vi "Autonomous Independent (2).vi"   [LabVIEW 2015]
doc: "This VI is called when autonomous begins, and will automatically be terminated when autonomous ends. You can carry out timed or sensor driven robot movement independently without needing to return to the caller."
uses:
  <vilib>/Rock Robotics/WPI/RobotDrive/WPI_RobotDriveArcadeDrive_Standard(NoSaturation).vi
  <vilib>/Rock Robotics/Network Tables/NT Write Numeric Array.vi
panel:
  # "Be sure to right-click and choose Data Operations>>Make Current Value default if you want to save the array values with the VI"
types:
  T1 = typedef "WPI_JoystickDevRef.ctl" = cluster{"Device":T2}
  T2 = typedef "WPI_JoystickDeviceEnum.ctl" = enum16{"USB 0", "USB 1", "USB 2", "USB 3", "USB 4", "USB 5"}
  T3 = typedef "WPI_DigitalInputDevRef.ctl" = cluster{"DevStatus":errorcluster, "DIO Channel":T4}
  T4 = typedef "FPGA_DIOChannel.ctl" = enum8{"DIO 0", "DIO 1", "DIO 2", "DIO 3", "DIO 4", "DIO 5", "DIO 6", "DIO 7", "DIO 8", "DIO 9", "DIO MXP 0", "DIO MXP 1", "DIO MXP 2", "DIO MXP 3", "DIO MXP 4", "DIO MXP 5", "DIO MXP 6", "DIO MXP 7", "DIO MXP 8", "DIO MXP 9", "DIO MXP 10", "DIO MXP 11", "DIO MXP 12", "DIO MXP 13", "DIO MXP 14", "DIO MXP 15", "Invalid"}
  T5 = typedef "WPI_MotorControlDeviceRef.ctl" = cluster{"DeviceStatus":errorcluster, "Type":T6, "PWM":cluster{"PWM Channel":T7, "DeadBand":T8}, "CAN":cluster{"Device Number":u8, "Control Mode":T9, "Semaphore":T10, "Max Vout":dbl, "TalonSRX Control Mode":T11}, "Invert":bool}
  T6 = typedef "WPI_MotorControlType.ctl" = enum16{"PWM", "CAN", "CANTalonSRX"}
  T7 = typedef "FPGA_DIOPWMChannel.ctl" = enum8{"PWM 0", "PWM 1", "PWM 2", "PWM 3", "PWM 4", "PWM 5", "PWM 6", "PWM 7", "PWM 8", "PWM 9", "PWM MXP 0", "PWM MXP 1", "PWM MXP 2", "PWM MXP 3", "PWM MXP 4", "PWM MXP 5", "PWM MXP 6", "PWM MXP 7", "PWM MXP 8", "PWM MXP 9", "Invalid"}
  T8 = typedef "WPI_PWMDeadband.ctl" = cluster{"Name":string, "maxPositivePwm":i32, "minPositivePwm":i32, "centerPwm":i32, "maxNegativePwm":i32, "minNegativePwm":i32, "angularRange":u16}
  T9 = typedef "WPI_CANJaguar_ControlMode.ctl" = enum8{"Percent VBus", "Current", "Speed", "Position", "Voltage"}
  T10 = typedef "Semaphore RefNum" = refnum<k1>
  T11 = typedef "WPI_CANTalonSRX_APIControlMode.ctl" = enum8{"Percent VBus", "Speed", "Position", "Slave", "Unchanged / Invalid", "Voltage Compensation", "Current", "Motion Profile"}
  T12 = typedef "WPI_GyroDevRef.ctl" = cluster{"DevStatus":errorcluster, "Analog Channel":T13, "Offset":dbl, "Gain (VoltsPerDegree/Second)":dbl, "Gyro Type":enum16{"Analog", "XRS450"}, "Handle":i32, "SPI Bus":T14, "Device Found":bool, "Sample Rate":dbl, "Calibrate On Open":bool}
  T13 = typedef "FPGA_AIChannel.ctl" = enum8{"AI 0", "AI 1", "AI 2", "AI 3", "AI MXP 0", "AI MXP 1", "AI MXP 2", "AI MXP 3", "Invalid"}
  T14 = typedef "spi_bus.ctl" = enum16{"SPI On-Board, CS0", "SPI On-Board, CS1", "SPI On-Board, CS2", "SPI On-Board, CS3", "SPI MXP", "Invalid"}
  T15 = typedef "WPI_CameraDevRef.ctl" = cluster{"Camera Address":string, "CameraStatus":errorcluster}
  T16 = typedef "WPI_AccelerometerDevRef.ctl" = cluster{"DevStatus":errorcluster, "Scaling":T17, "Analog Channels":T18, "I2C Bus":T19, "SPI Bus":T14, "Accel Range":T20, "ADXL Axes":T21, "Handle":i32, "Device Address":u8, "Accel Type":enum16{"Analog", "ADXL345 I2C", "ADXL345 SPI", "Internal", "ADXL362 SPI"}}
  T17 = typedef "WPI_AccelerometerScaling.ctl" = cluster{"Gain (VoltsPerG)":dbl, "Center Voltage":dbl}
  T18 = typedef "WPI_AccelerometerAnalogChannels.ctl" = cluster{"X-Axis":T13, "Y-Axis":T13, "Z-Axis":T13}
  T19 = typedef "i2c_bus.ctl" = enum16{"I2C On-Board", "I2C MXP", "Invalid"}
  T20 = typedef "ADXL345 Range.ctl" = u8
  T21 = typedef "WPI_AccelerometerADXL345 Axes.ctl" = cluster{"X-Axis":bool, "Y-Axis":bool, "Z-Axis":bool}
  T22 = typedef "WPI_EncoderDevRef.ctl" = cluster{"DevStatus":errorcluster, "EncoderIndex":T23, "CounterIndex":T24, "DistancePerCount":dbl, "Decoding Type":T25}
  T23 = typedef "FPGA_EncoderIdx.ctl" = enum8{"Enc 0", "Enc 1", "Enc 2", "Enc 3", "Enc 4", "Enc 5", "Enc 6", "Enc 7", "Invalid"}
  T24 = typedef "FPGA_CounterCtrSystemIndex.ctl" = enum8{"Ctr 0", "Ctr 1", "Ctr 2", "Ctr 3", "Ctr 4", "Ctr 5", "Ctr 6", "Ctr 7", "Invalid"}
  T25 = typedef "WPI_EncoderType.ctl" = enum16{"1x", "2x", "4x"}
  T26 = typedef "WPI_RobotDriveDevRef.ctl" = cluster{"DevStatus":errorcluster, "Motors[]":T5[], "Square Inputs":bool, "Max Output":dbl}
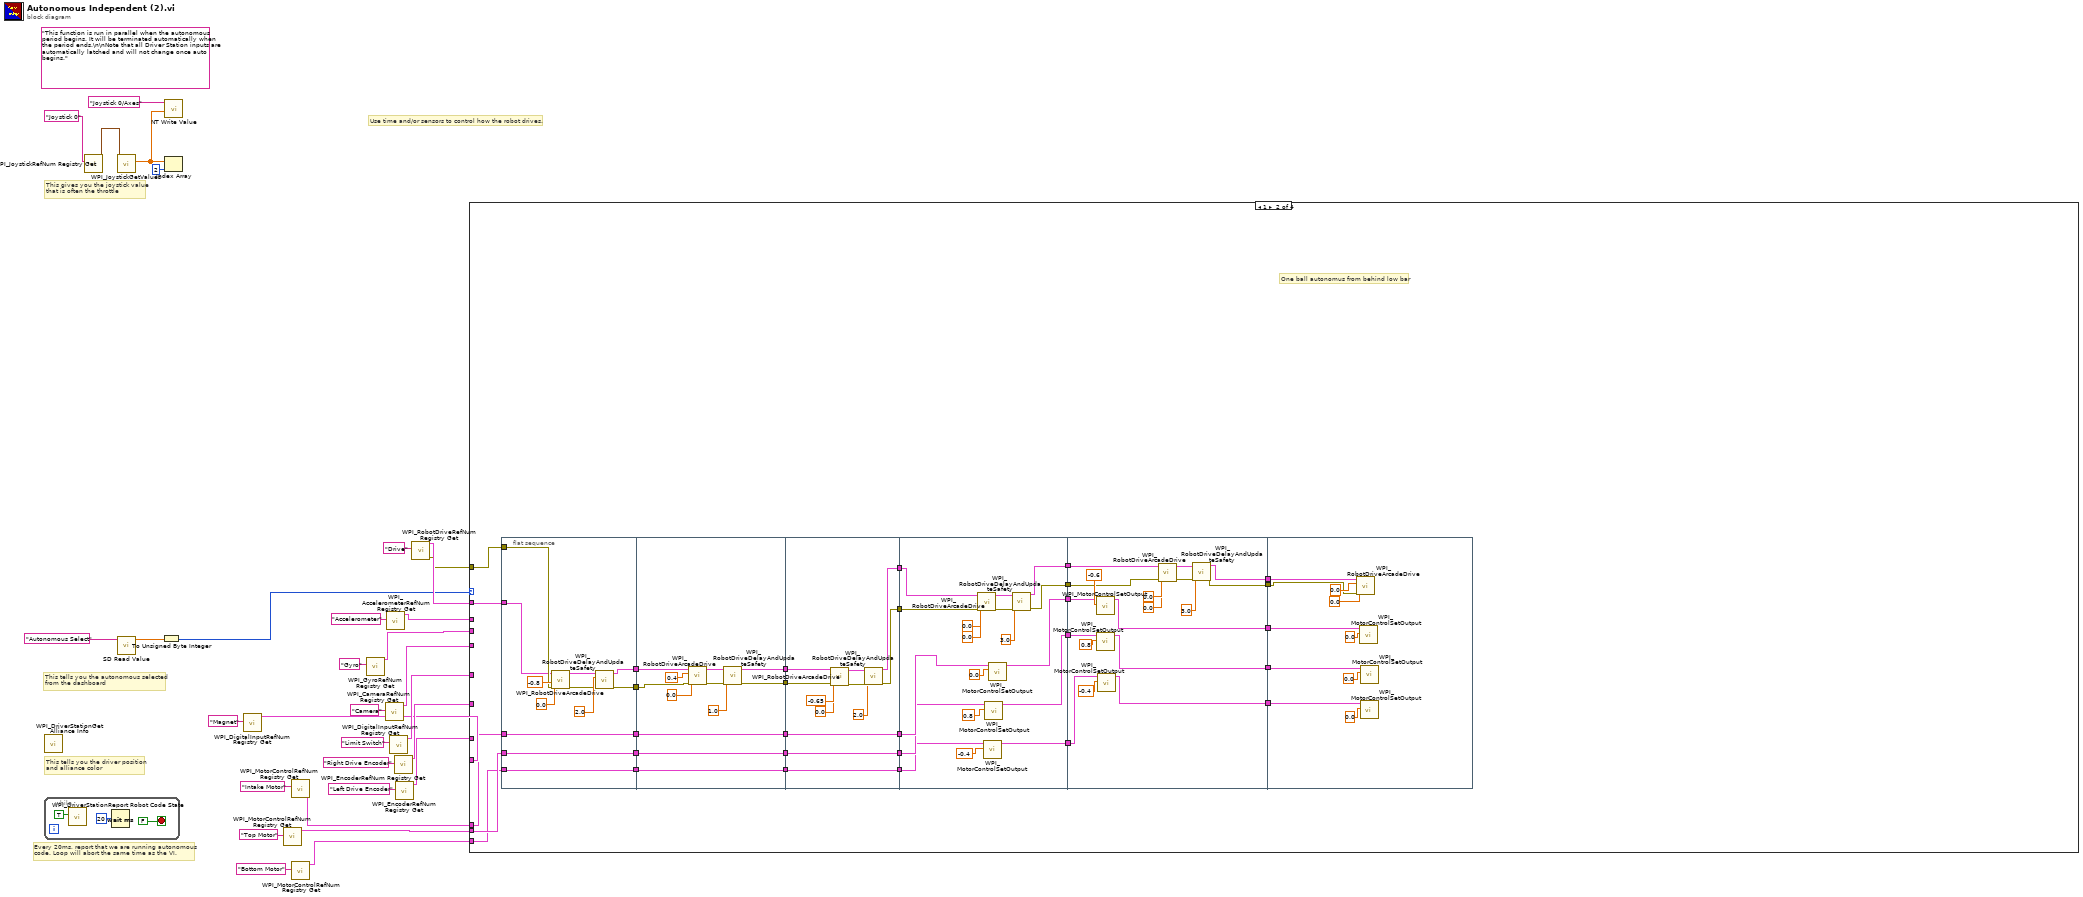
[diagram p0: block diagram]
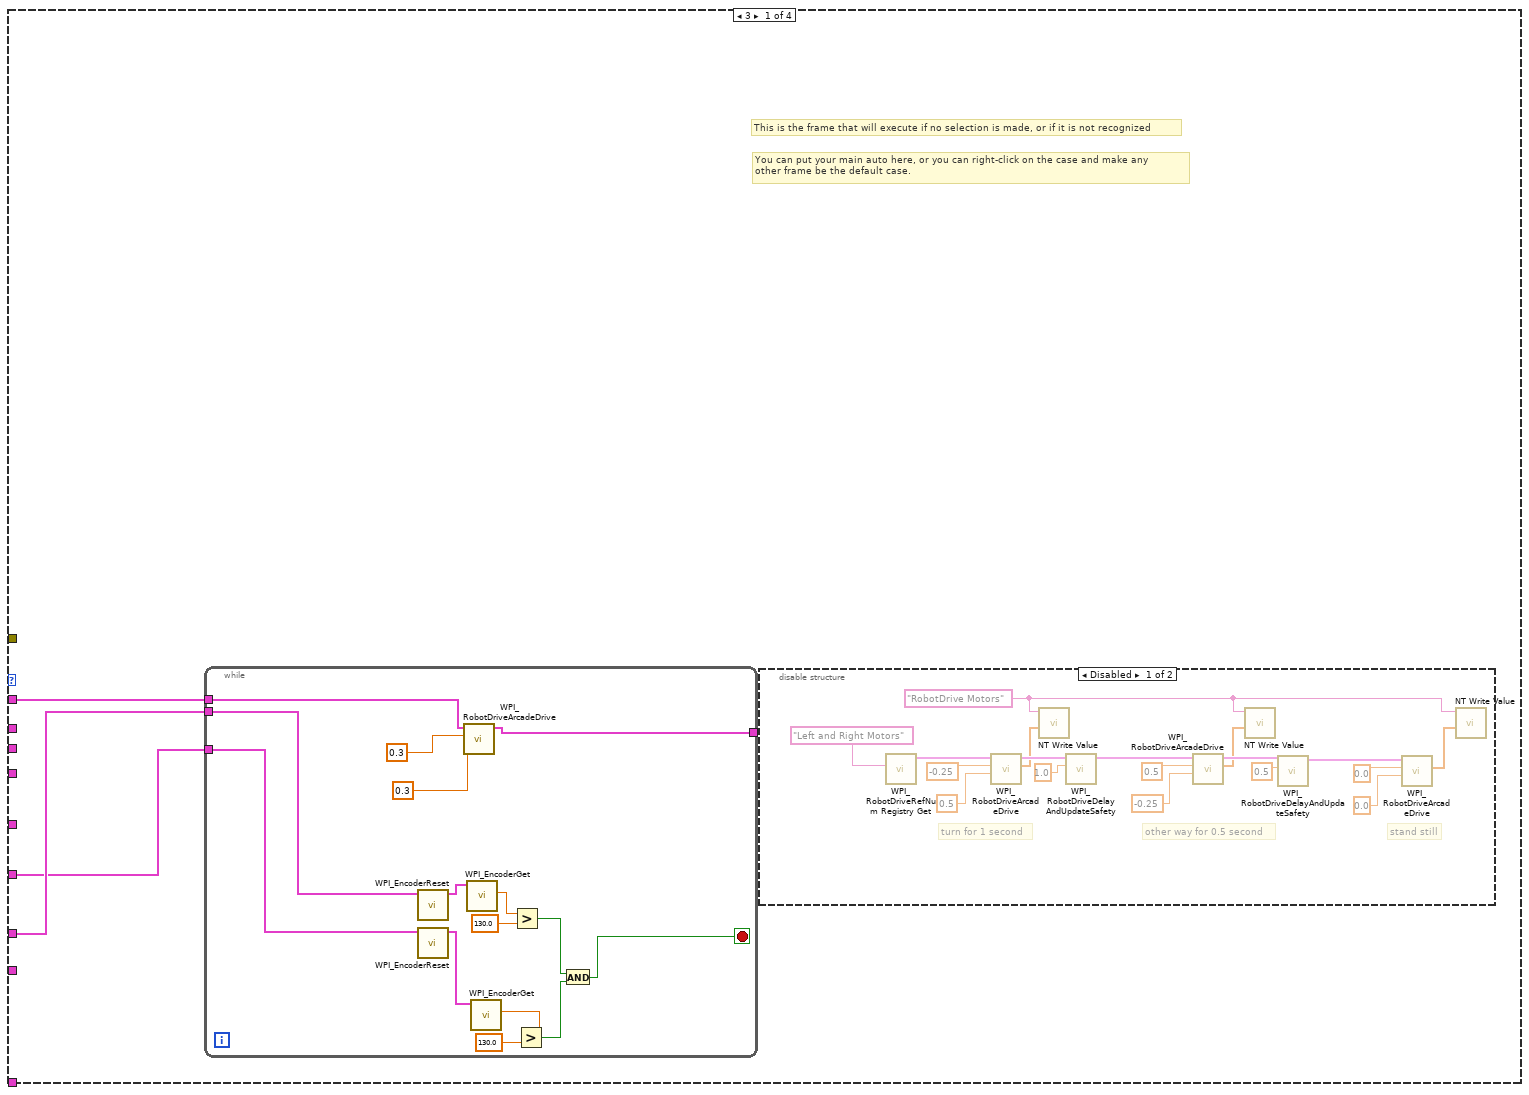
[diagram p2: hidden frame]
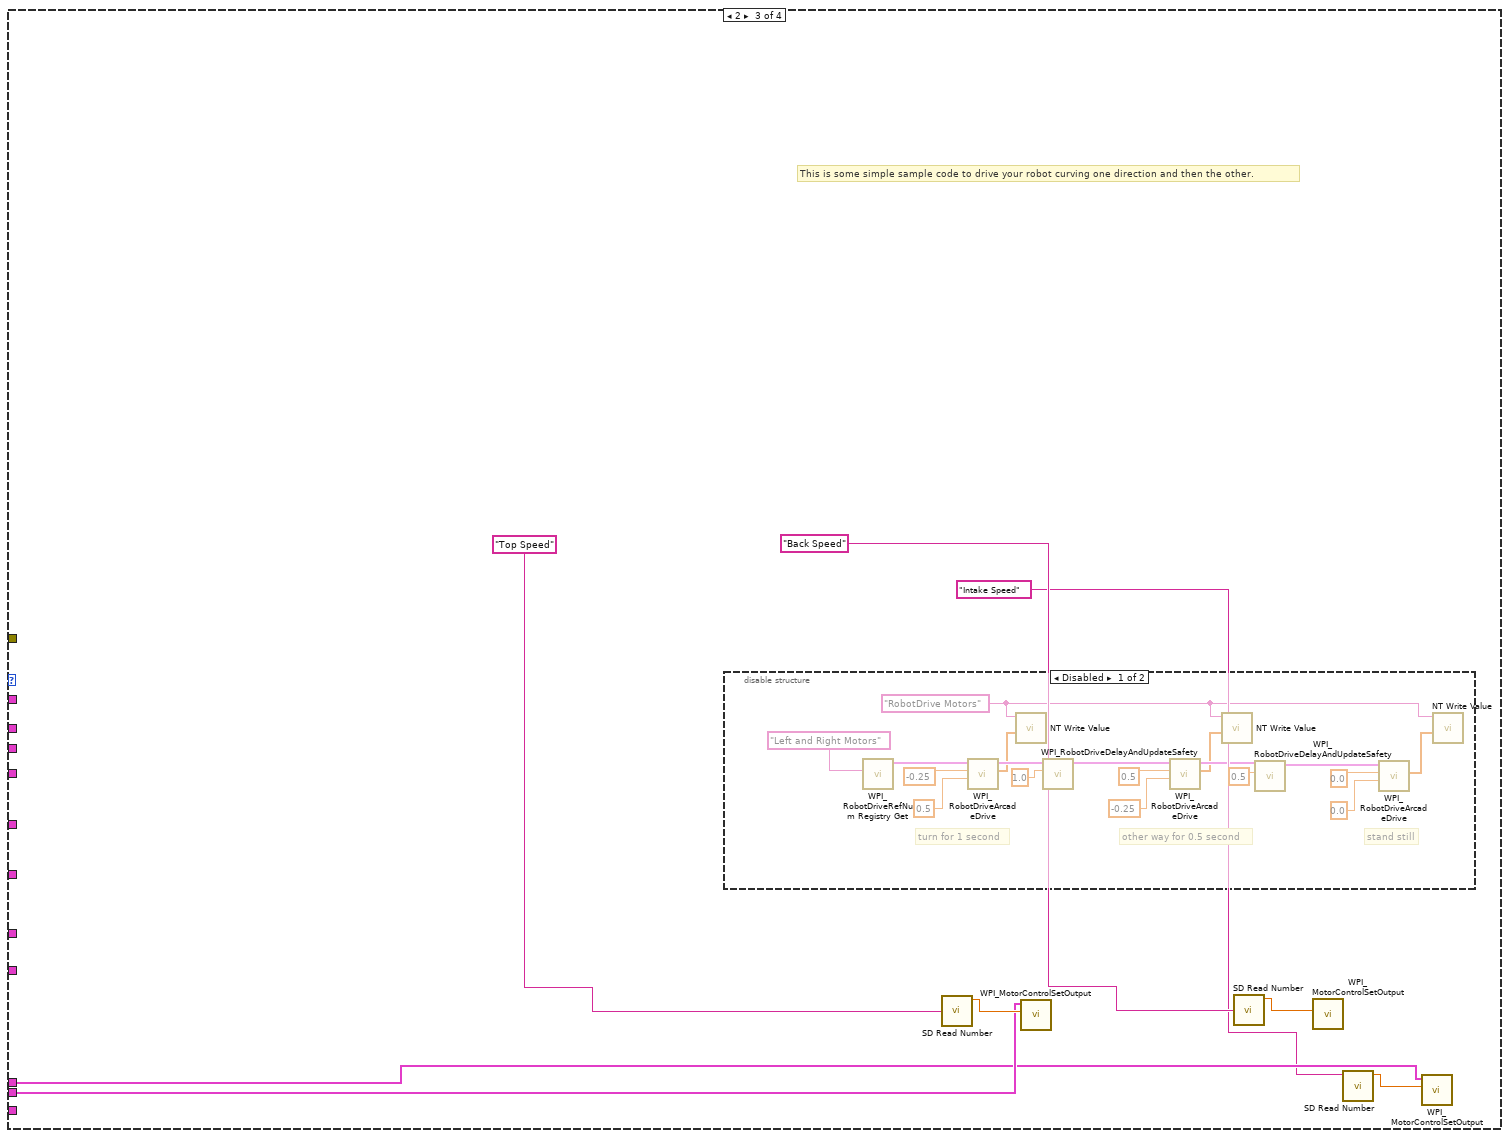
[diagram p4: hidden frame]
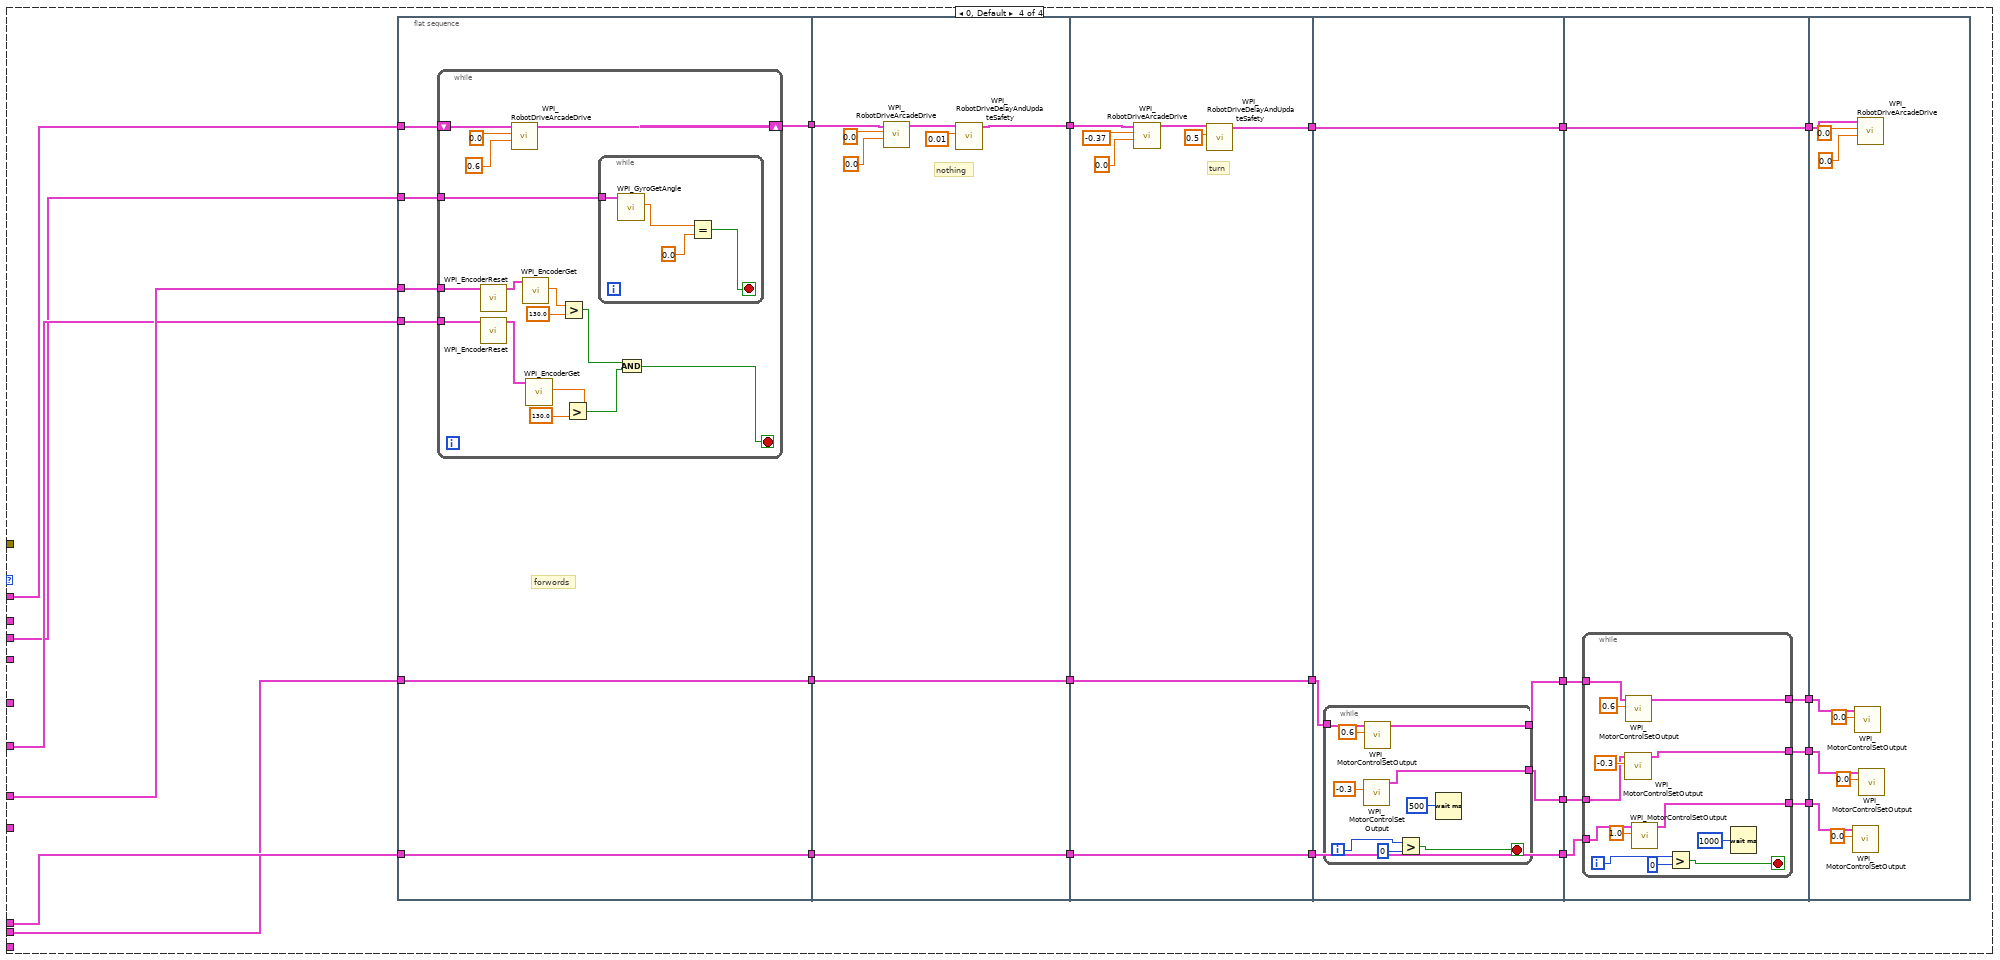
[diagram p6: hidden frame]
diagram:
  (unwired) "This function is run in parallel when the autonomous period begins. It will be terminated automatically when the period ends.\n\nNote that all Driver Station inputs are automatically latched and will not change once auto begins."
  # "This tells you the autonomous selected\nfrom the dashboard"
  # "Every 20ms, report that we are running autonomous\ncode. Loop will abort the same time as the VI."
  # "This tells you the driver position\nand alliance color"
  # "Use time and/or sensors to control how the robot drives."
  # "This gives you the joystick value\nthat is often the throttle"
  n1 = while {
    stop <- FALSE stop-if-true
    n2 = call <vilib>:"WPI_DriverStationReport Robot Code State.vi"("Autonomous"=TRUE) -> ()  [unwired: 10 in, 1 out]
    n3 = Wait (ms)(milliseconds to wait=u32 20) -> ()  [unwired: 1 out]
  }
  n4 = call <vilib>:"WPI_DriverStationGet Alliance Info.vi"() -> ()  [unwired: 12 out]
  n5 = call <vilib>:"WPI_JoystickRefNum Registry Get.vi"("refnum name"="Joystick 0") -> ("JoystickDevRef"=w30:T1)  [unwired: 1 in, 9 out]
  n6 = call <vilib>:"WPI_JoystickGetValues.vi"("JoystickDevRef"=w30) -> ("Axes"=w28:dbl[])  [unwired: 6 in, 4 out]
  n7 = call-poly <vilib>:"SD Read Value.vi"("Name"="Autonomous Select") -> ("Numeric"=w16:dbl)  [unwired: 8 in, 2 out]
  n8 = To Unsigned Byte Integer(number=w16) -> (unsigned 8bit integer=w14:u8)
  n9 = call-poly <vilib>:"NT Write Value.vi"("Numeric Array"=w28, "Name"="Joystick 0/Axes") -> ()  [unwired: 9 in, 1 out]
  n10 = Index Array(array=w28, index=2) -> ()  [unwired: 1 out]
  n11 = call <vilib>:"WPI_DigitalInputRefNum Registry Get.vi"("refnum name"="Magnet") -> ("DigitalInputDevRef"=w17:T3)  [unwired: 9 in, 1 out]
  n12 = call <vilib>:"WPI_MotorControlRefNum Registry Get.vi"("refnum name"="Top Motor") -> ("MotorControlDevRef"=w3:T5)  [unwired: 9 in, 1 out]
  n13 = call <vilib>:"WPI_MotorControlRefNum Registry Get.vi"("refnum name"="Intake Motor") -> ("MotorControlDevRef"=w11:T5)  [unwired: 9 in, 1 out]
  n14 = call <vilib>:"WPI_MotorControlRefNum Registry Get.vi"("refnum name"="Bottom Motor") -> ("MotorControlDevRef"=w1:T5)  [unwired: 9 in, 1 out]
  n15 = call <vilib>:"WPI_GyroRefNum Registry Get.vi"("refnum name"="Gyro") -> ("GyroDevRef"=w22:T12)  [unwired: 9 in, 1 out]
  n16 = call <vilib>:"WPI_CameraRefNum Registry Get.vi"("refnum name"="Camera") -> ("CameraDevRef"=w21:T15)  [unwired: 9 in, 1 out]
  n17 = call <vilib>:"WPI_AccelerometerRefNum Registry Get.vi"("refnum name"="Accelerometer") -> ("AccelerometerDevRef"=w23:T16)  [unwired: 9 in, 1 out]
  n18 = call <vilib>:"WPI_DigitalInputRefNum Registry Get.vi"("refnum name"="Limit Switch") -> ("DigitalInputDevRef"=w20:T3)  [unwired: 9 in, 1 out]
  n19 = call <vilib>:"WPI_EncoderRefNum Registry Get.vi"("refnum name"="Right Drive Encoder") -> ("EncoderDevRef"=w19:T22)  [unwired: 9 in, 1 out]
  n20 = call <vilib>:"WPI_EncoderRefNum Registry Get.vi"("refnum name"="Left Drive Encoder") -> ("EncoderDevRef"=w18:T22)  [unwired: 9 in, 1 out]
  n21 = call <vilib>:"WPI_RobotDriveRefNum Registry Get.vi"("refnum name"="Drive") -> ("error out"=w2:errorcluster, "RobotDriveDevRef"=w26:T26)  [unwired: 9 in]
  n22 = case shown="1" w14 {
    tunnel: w26 -> [w35 w83 _ w213]
    tunnel: w23 -> [_ _ _ _]
    tunnel: w22 -> [_ _ _ w209]
    tunnel: w21 -> [_ _ _ _]
    tunnel: w20 -> [_ _ _ _]
    tunnel: w19 -> [w36 _ _ w210]
    tunnel: w18 -> [w37 _ _ w211]
    tunnel: w17 -> [_ _ _ _]
    tunnel: w3 -> [_ w78 w188 w214]
    tunnel: w11 -> [_ w82 w185 w215]
    tunnel: w2 -> [_ w85 _ _]
    tunnel: w1 -> [_ w71 _ _]
    frame 3 {
      # "You can put your main auto here, or you can right-click on the case and make any\nother frame be the default case."
      # "This is the frame that will execute if no selection is made, or if it is not recognized"
      n23 = while {
        tunnel: w37 -> [w46]
        tunnel: w36 -> [w45]
        tunnel: w35 -> [w41]
        tunnel: [w40] -> _
        stop <- w42 stop-if-true
        n24 = call <vilib>:"WPI_EncoderReset.vi"("EncoderDevRef"=w46) -> ("EncoderDevRef"=w48:T22)  [unwired: 9 in, 1 out]
        n25 = call <vilib>:"WPI_EncoderReset.vi"("EncoderDevRef"=w45) -> ("EncoderDevRef"=w52:T22)  [unwired: 9 in, 1 out]
        n26 = call-poly <vilib>:"WPI_RobotDriveArcadeDrive.vi"("Y axis value"=0.3, "X axis value"=0.3, "RobotDriveDevRef"=w41) -> ("RobotDriveDevRef"=w40:T26)  [unwired: 6 in, 2 out]
        n27 = call <vilib>:"WPI_EncoderGet.vi"("EncoderDevRef"=w48) -> ("Distance"=w49:dbl)  [unwired: 5 in, 5 out]
        n28 = call <vilib>:"WPI_EncoderGet.vi"("EncoderDevRef"=w52) -> ("Distance"=w51:dbl)  [unwired: 5 in, 5 out]
        n29 = Greater?(x=w49, y=130.0) -> (0:w44:bool)
        n30 = Greater?(x=w51, y=130.0) -> (0:w43:bool)
        n31 = And(x=w44, y=w43) -> (x .and. y?=w42:bool)
      }
      n32 = disable-structure shown="Disabled" {
        frame Disabled {
          w54 = "RobotDrive Motors" ("Name")
          # "stand still"
          # "other way for 0.5 second"
          # "turn for 1 second"
          n33 = call <vilib>:"WPI_RobotDriveRefNum Registry Get.vi"("refnum name"="Left and Right Motors") -> ("RobotDriveDevRef"=w70:T26)  [unwired: 1 in, 9 out]
          n34 = call-poly <vilib>:"WPI_RobotDriveArcadeDrive.vi"("Y axis value"=0.5 ("X axis value"), "X axis value"=-0.25, "RobotDriveDevRef"=w70) -> ("Motor Values"=w53:dbl[], "RobotDriveDevRef"=w63:T26)  [unwired: 1 in, 6 out]
          n35 = call-poly <vilib>:"NT Write Value.vi"("Numeric Array"=w53, "Name"=w54) -> ()  [unwired: 9 in, 1 out]
          n36 = call <vilib>:"WPI_RobotDriveDelayAndUpdateSafety.vi"("Delay (s)"=1.0, "RobotDriveDevRef"=w63) -> ("RobotDriveDevRef 2"=w64:T26)  [unwired: 8 in, 1 out]
          n37 = call-poly <vilib>:"WPI_RobotDriveArcadeDrive.vi"("Y axis value"=-0.25 ("X axis value"), "X axis value"=0.5, "RobotDriveDevRef"=w64) -> ("Motor Values"=w55:dbl[], "RobotDriveDevRef"=w65:T26)  [unwired: 1 in, 6 out]
          n38 = call-poly <vilib>:"NT Write Value.vi"("Numeric Array"=w55, "Name"=w54) -> ()  [unwired: 9 in, 1 out]
          n39 = call <vilib>:"WPI_RobotDriveDelayAndUpdateSafety.vi"("Delay (s)"=0.5, "RobotDriveDevRef"=w65) -> ("RobotDriveDevRef 2"=w66:T26)  [unwired: 8 in, 1 out]
          n40 = call-poly <vilib>:"WPI_RobotDriveArcadeDrive.vi"("Y axis value"=0.0 ("X axis value"), "X axis value"=0.0, "RobotDriveDevRef"=w66) -> ("Motor Values"=w56:dbl[])  [unwired: 1 in, 7 out]
          n41 = call-poly <vilib>:"NT Write Value.vi"("Numeric Array"=w56, "Name"=w54) -> ()  [unwired: 9 in, 1 out]
        }
        frame Enabled {
        }
      }
    }
    frame 1 {
      # "One ball autonomus from behind low bar"
      n42 = flat-sequence {
        tunnel: [w107] -> w100
        tunnel: [w106] -> w86
        tunnel: w85 -> [w105]
        tunnel: w83 -> [w104]
        tunnel: w82 -> [w103]
        tunnel: [w103] -> w79
        tunnel: w78 -> [w102]
        tunnel: [w102] -> w75
        tunnel: w71 -> [w101]
        tunnel: [w101] -> w72
        tunnel: w100 -> [w119]
        tunnel: [w118] -> w99
        tunnel: [w117] -> w89
        tunnel: w86 -> [w116]
        tunnel: [w115] -> w80
        tunnel: w79 -> [w115]
        tunnel: [w114] -> w76
        tunnel: w75 -> [w114]
        tunnel: [w113] -> w73
        tunnel: w72 -> [w113]
        tunnel: w99 -> [w133]
        tunnel: [w132] -> w98
        tunnel: w89 -> [w129]
        tunnel: [w128] -> w88
        tunnel: [w127] -> w81
        tunnel: w80 -> [w127]
        tunnel: [w126] -> w77
        tunnel: w76 -> [w126]
        tunnel: [w125] -> w74
        tunnel: w73 -> [w125]
        tunnel: w98 -> [w150]
        tunnel: [w148] -> w94
        tunnel: [w147] -> w93
        tunnel: [w146] -> w91
        tunnel: [w145] -> w90
        tunnel: w88 -> [w144]
        tunnel: [w143] -> w87
        tunnel: w81 -> [w142]
        tunnel: w77 -> [w141]
        tunnel: w74 -> [w140]
        tunnel: [w172] -> w97
        tunnel: [w171] -> w96
        tunnel: [w170] -> w95
        tunnel: w94 -> [w166]
        tunnel: w93 -> [w160]
        tunnel: [w159] -> w92
        tunnel: w91 -> [w158]
        tunnel: w90 -> [w157]
        tunnel: w87 -> [w156]
        tunnel: [w155] -> w84
        tunnel: w97 -> [w182]
        tunnel: w96 -> [w181]
        tunnel: w95 -> [w180]
        tunnel: w92 -> [w174]
        tunnel: w84 -> [w173]
        frame #0 {
          n43 = call-poly <vilib>:"WPI_RobotDriveArcadeDrive.vi"("error in (no error)"=w105, "Y axis value"=-0.8, "X axis value"=0.0, "RobotDriveDevRef"=w104) -> ("error out"=w109:errorcluster, "RobotDriveDevRef"=w108:T26)  [unwired: 5 in, 1 out]
          n44 = call <vilib>:"WPI_RobotDriveDelayAndUpdateSafety.vi"("error in (no error)"=w109, "Delay (s)"=2.0, "RobotDriveDevRef"=w108) -> ("error out"=w106:errorcluster, "RobotDriveDevRef 2"=w107:T26)  [unwired: 7 in]
        }
        frame #1 {
          n45 = call-poly <vilib>:"WPI_RobotDriveArcadeDrive.vi"("error in (no error)"=w116, "Y axis value"=0.0, "X axis value"=0.4, "RobotDriveDevRef"=w119) -> ("error out"=w121:errorcluster, "RobotDriveDevRef"=w122:T26)  [unwired: 5 in, 1 out]
          n46 = call <vilib>:"WPI_RobotDriveDelayAndUpdateSafety.vi"("error in (no error)"=w121, "Delay (s)"=1.0, "RobotDriveDevRef"=w122) -> ("error out"=w117:errorcluster, "RobotDriveDevRef 2"=w118:T26)  [unwired: 7 in]
        }
        frame #2 {
          n47 = call-poly <vilib>:"WPI_RobotDriveArcadeDrive.vi"("error in (no error)"=w129, "Y axis value"=-0.65, "X axis value"=0.0, "RobotDriveDevRef"=w133) -> ("error out"=w136:errorcluster, "RobotDriveDevRef"=w135:T26)  [unwired: 5 in, 1 out]
          n48 = call <vilib>:"WPI_RobotDriveDelayAndUpdateSafety.vi"("error in (no error)"=w136, "Delay (s)"=2.0, "RobotDriveDevRef"=w135) -> ("error out"=w128:errorcluster, "RobotDriveDevRef 2"=w132:T26)  [unwired: 7 in]
        }
        frame #3 {
          n49 = call-poly <vilib>:"WPI_RobotDriveArcadeDrive.vi"("error in (no error)"=w144, "Y axis value"=0.0, "X axis value"=0.0, "RobotDriveDevRef"=w150) -> ("error out"=w151:errorcluster, "RobotDriveDevRef"=w149:T26)  [unwired: 5 in, 1 out]
          n50 = call <vilib>:"WPI_MotorControlSetOutput.vi"("Output"=-0.4, "MotorControlDevRef"=w140) -> ("MotorControlDevRef"=w145:T5)  [unwired: 7 in, 2 out]
          n51 = call <vilib>:"WPI_MotorControlSetOutput.vi"("Output"=0.8, "MotorControlDevRef"=w141) -> ("MotorControlDevRef"=w146:T5)  [unwired: 7 in, 2 out]
          n52 = call <vilib>:"WPI_MotorControlSetOutput.vi"("Output"=0.0, "MotorControlDevRef"=w142) -> ("MotorControlDevRef"=w148:T5)  [unwired: 7 in, 2 out]
          n53 = call <vilib>:"WPI_RobotDriveDelayAndUpdateSafety.vi"("error in (no error)"=w151, "Delay (s)"=3.0, "RobotDriveDevRef"=w149) -> ("error out"=w143:errorcluster, "RobotDriveDevRef 2"=w147:T26)  [unwired: 7 in]
        }
        frame #4 {
          n54 = call <vilib>:"WPI_MotorControlSetOutput.vi"("Output"=-0.6, "MotorControlDevRef"=w166) -> ("MotorControlDevRef"=w172:T5)  [unwired: 7 in, 2 out]
          n55 = call <vilib>:"WPI_MotorControlSetOutput.vi"("Output"=0.8, "MotorControlDevRef"=w158) -> ("MotorControlDevRef"=w171:T5)  [unwired: 7 in, 2 out]
          n56 = call <vilib>:"WPI_MotorControlSetOutput.vi"("Output"=-0.4, "MotorControlDevRef"=w157) -> ("MotorControlDevRef"=w170:T5)  [unwired: 7 in, 2 out]
          n57 = call-poly <vilib>:"WPI_RobotDriveArcadeDrive.vi"("error in (no error)"=w156, "Y axis value"=0.0, "X axis value"=0.0, "RobotDriveDevRef"=w160) -> ("error out"=w164:errorcluster, "RobotDriveDevRef"=w165:T26)  [unwired: 5 in, 1 out]
          n58 = call <vilib>:"WPI_RobotDriveDelayAndUpdateSafety.vi"("error in (no error)"=w164, "Delay (s)"=3.0, "RobotDriveDevRef"=w165) -> ("error out"=w155:errorcluster, "RobotDriveDevRef 2"=w159:T26)  [unwired: 7 in]
        }
        frame #5 {
          n59 = call-poly <vilib>:"WPI_RobotDriveArcadeDrive.vi"("error in (no error)"=w173, "Y axis value"=0.0, "X axis value"=0.0, "RobotDriveDevRef"=w174) -> ()  [unwired: 5 in, 3 out]
          n60 = call <vilib>:"WPI_MotorControlSetOutput.vi"("Output"=0.0, "MotorControlDevRef"=w182) -> ()  [unwired: 7 in, 3 out]
          n61 = call <vilib>:"WPI_MotorControlSetOutput.vi"("Output"=0.0, "MotorControlDevRef"=w180) -> ()  [unwired: 7 in, 3 out]
          n62 = call <vilib>:"WPI_MotorControlSetOutput.vi"("Output"=0.0, "MotorControlDevRef"=w181) -> ()  [unwired: 7 in, 3 out]
        }
      }
    }
    frame 2 {
      # "This is some simple sample code to drive your robot curving one direction and then the other."
      n63 = disable-structure shown="Disabled" {
        frame Disabled {
          w192 = "RobotDrive Motors" ("Name")
          # "stand still"
          # "other way for 0.5 second"
          # "turn for 1 second"
          n64 = call <vilib>:"WPI_RobotDriveRefNum Registry Get.vi"("refnum name"="Left and Right Motors") -> ("RobotDriveDevRef"=w208:T26)  [unwired: 1 in, 9 out]
          n65 = call-poly <vilib>:"WPI_RobotDriveArcadeDrive.vi"("Y axis value"=0.5 ("X axis value"), "X axis value"=-0.25, "RobotDriveDevRef"=w208) -> ("Motor Values"=w191:dbl[], "RobotDriveDevRef"=w201:T26)  [unwired: 1 in, 6 out]
          n66 = call-poly <vilib>:"NT Write Value.vi"("Numeric Array"=w191, "Name"=w192) -> ()  [unwired: 9 in, 1 out]
          n67 = call <vilib>:"WPI_RobotDriveDelayAndUpdateSafety.vi"("Delay (s)"=1.0, "RobotDriveDevRef"=w201) -> ("RobotDriveDevRef 2"=w202:T26)  [unwired: 8 in, 1 out]
          n68 = call-poly <vilib>:"WPI_RobotDriveArcadeDrive.vi"("Y axis value"=-0.25 ("X axis value"), "X axis value"=0.5, "RobotDriveDevRef"=w202) -> ("Motor Values"=w193:dbl[], "RobotDriveDevRef"=w203:T26)  [unwired: 1 in, 6 out]
          n69 = call-poly <vilib>:"NT Write Value.vi"("Numeric Array"=w193, "Name"=w192) -> ()  [unwired: 9 in, 1 out]
          n70 = call <vilib>:"WPI_RobotDriveDelayAndUpdateSafety.vi"("Delay (s)"=0.5, "RobotDriveDevRef"=w203) -> ("RobotDriveDevRef 2"=w204:T26)  [unwired: 8 in, 1 out]
          n71 = call-poly <vilib>:"WPI_RobotDriveArcadeDrive.vi"("Y axis value"=0.0 ("X axis value"), "X axis value"=0.0, "RobotDriveDevRef"=w204) -> ("Motor Values"=w194:dbl[])  [unwired: 1 in, 7 out]
          n72 = call-poly <vilib>:"NT Write Value.vi"("Numeric Array"=w194, "Name"=w192) -> ()  [unwired: 9 in, 1 out]
        }
        frame Enabled {
        }
      }
      n73 = call <vilib>:"SD Read Number.vi"("Name"="Top Speed" ("refnum name")) -> ("Numeric"=w189:dbl)  [unwired: 8 in, 2 out]
      n74 = call <vilib>:"WPI_MotorControlSetOutput.vi"("Output"=w189, "MotorControlDevRef"=w188) -> ()  [unwired: 7 in, 3 out]
      n75 = call <vilib>:"SD Read Number.vi"("Name"="Back Speed" ("refnum name")) -> ("Numeric"=w186:dbl)  [unwired: 8 in, 2 out]
      n76 = call <vilib>:"WPI_MotorControlSetOutput.vi"("Output"=w186) -> ()  [unwired: 8 in, 3 out]
      n77 = call <vilib>:"SD Read Number.vi"("Name"="Intake Speed") -> ("Numeric"=w184:dbl)  [unwired: 8 in, 2 out]
      n78 = call <vilib>:"WPI_MotorControlSetOutput.vi"("Output"=w184, "MotorControlDevRef"=w185) -> ()  [unwired: 7 in, 3 out]
    }
    frame 0, Default {
      n79 = flat-sequence {
        tunnel: w213 -> [w238]
        tunnel: w214 -> [w237]
        tunnel: [w237] -> w231
        tunnel: w215 -> [w236]
        tunnel: [w236] -> w230
        tunnel: [w235] -> w212
        tunnel: w211 -> [w234]
        tunnel: w210 -> [w233]
        tunnel: w209 -> [w232]
        tunnel: [w262] -> w229
        tunnel: w231 -> [w261]
        tunnel: [w261] -> w228
        tunnel: [w260] -> w227
        tunnel: w230 -> [w260]
        tunnel: w212 -> [w259]
        tunnel: w229 -> [w270]
        tunnel: w228 -> [w269]
        tunnel: [w269] -> w226
        tunnel: [w268] -> w225
        tunnel: w227 -> [w268]
        tunnel: [w267] -> w224
        tunnel: w226 -> [w279]
        tunnel: w225 -> [w278]
        tunnel: [w278] -> w223
        tunnel: [w277] -> w222
        tunnel: [w276] -> w221
        tunnel: [w275] -> w220
        tunnel: w224 -> [w275]
        tunnel: w223 -> [w292]
        tunnel: w222 -> [w294]
        tunnel: w221 -> [w293]
        tunnel: [w295] -> w219
        tunnel: w220 -> [w295]
        tunnel: [w291] -> w218
        tunnel: [w290] -> w217
        tunnel: [w289] -> w216
        tunnel: w219 -> [w315]
        tunnel: w218 -> [w314]
        tunnel: w217 -> [w313]
        tunnel: w216 -> [w312]
        frame #0 {
          # "forwords"
          n80 = while {
            shift-right: [w254] -> w235
            shift-left: w238 -> [w251]
            tunnel: w234 -> [w250]
            tunnel: w233 -> [w249]
            tunnel: w232 -> [w239]
            stop <- w240 stop-if-true
            n81 = call <vilib>:"WPI_EncoderReset.vi"("EncoderDevRef"=w250) -> ("EncoderDevRef"=w247:T22)  [unwired: 9 in, 1 out]
            n82 = call <vilib>:"WPI_EncoderReset.vi"("EncoderDevRef"=w249) -> ("EncoderDevRef"=w243:T22)  [unwired: 9 in, 1 out]
            n83 = call-poly <vilib>:"WPI_RobotDriveArcadeDrive.vi"("Y axis value"=0.6 ("X axis value"), "X axis value"=0.0, "RobotDriveDevRef"=w251) -> ("RobotDriveDevRef"=w254:T26)  [unwired: 1 in, 7 out]
            n84 = call <vilib>:"WPI_EncoderGet.vi"("EncoderDevRef"=w247) -> ("Distance"=w246:dbl)  [unwired: 5 in, 5 out]
            n85 = call <vilib>:"WPI_EncoderGet.vi"("EncoderDevRef"=w243) -> ("Distance"=w244:dbl)  [unwired: 5 in, 5 out]
            n86 = Greater?(x=w246, y=130.0) -> (0:w241:bool)
            n87 = Greater?(x=w244, y=130.0) -> (0:w242:bool)
            n88 = while {
              tunnel: w239 -> [w258]
              stop <- w255 stop-if-true
              n89 = call <vilib>:"WPI_GyroGetAngle.vi"("GyroDevRef"=w258) -> ("Angle"=w257:dbl)  [unwired: 6 in, 4 out]
              n90 = Equal?(x=w257, y=0.0) -> (x = y?=w255:bool)
            }
            n91 = And(x=w241, y=w242) -> (x .and. y?=w240:bool)
          }
        }
        frame #1 {
          # "nothing"
          n92 = call-poly <vilib>:"WPI_RobotDriveArcadeDrive.vi"("Y axis value"=0.0 ("X axis value"), "X axis value"=0.0, "RobotDriveDevRef"=w259) -> ("RobotDriveDevRef"=w265:T26)  [unwired: 1 in, 7 out]
          n93 = call <vilib>:"WPI_RobotDriveDelayAndUpdateSafety.vi"("Delay (s)"=0.01, "RobotDriveDevRef"=w265) -> ("RobotDriveDevRef 2"=w262:T26)  [unwired: 8 in, 1 out]
        }
        frame #2 {
          # "turn"
          n94 = call-poly <vilib>:"WPI_RobotDriveArcadeDrive.vi"("Y axis value"=0.0 ("X axis value"), "X axis value"=-0.37, "RobotDriveDevRef"=w270) -> ("RobotDriveDevRef"=w273:T26)  [unwired: 1 in, 7 out]
          n95 = call <vilib>:"WPI_RobotDriveDelayAndUpdateSafety.vi"("Delay (s)"=0.5, "RobotDriveDevRef"=w273) -> ("RobotDriveDevRef 2"=w267:T26)  [unwired: 8 in, 1 out]
        }
        frame #3 {
          n96 = while {
            tunnel: w279 -> [w288]
            tunnel: [w285] -> w277
            tunnel: [w284] -> w276
            i -> [w281]
            stop <- w280 stop-if-true
            n97 = call <vilib>:"WPI_MotorControlSetOutput.vi"("Output"=-0.3) -> ("MotorControlDevRef"=w284:T5)  [unwired: 8 in, 2 out]
            n98 = call <vilib>:"WPI_MotorControlSetOutput.vi"("Output"=0.6, "MotorControlDevRef"=w288) -> ("MotorControlDevRef"=w285:T5)  [unwired: 7 in, 2 out]
            n99 = Greater?(x=w281, y=0) -> (0:w280:bool)
            n100 = Wait (ms)(milliseconds to wait=500) -> ()  [unwired: 1 out]
          }
        }
        frame #4 {
          n101 = while {
            tunnel: w294 -> [w306]
            tunnel: w293 -> [w305]
            tunnel: w292 -> [w304]
            tunnel: [w302] -> w291
            tunnel: [w301] -> w290
            tunnel: [w300] -> w289
            i -> [w298]
            stop <- w296 stop-if-true
            n102 = call <vilib>:"WPI_MotorControlSetOutput.vi"("Output"=-0.3, "MotorControlDevRef"=w305) -> ("MotorControlDevRef"=w301:T5)  [unwired: 7 in, 2 out]
            n103 = call <vilib>:"WPI_MotorControlSetOutput.vi"("Output"=0.6, "MotorControlDevRef"=w306) -> ("MotorControlDevRef"=w302:T5)  [unwired: 7 in, 2 out]
            n104 = call <vilib>:"WPI_MotorControlSetOutput.vi"("Output"=1.0, "MotorControlDevRef"=w304) -> ("MotorControlDevRef"=w300:T5)  [unwired: 7 in, 2 out]
            n105 = Greater?(x=w298, y=0) -> (0:w296:bool)
            n106 = Wait (ms)(milliseconds to wait=u32 1000) -> ()  [unwired: 1 out]
          }
        }
        frame #5 {
          n107 = call <vilib>:"WPI_MotorControlSetOutput.vi"("Output"=0.0, "MotorControlDevRef"=w312) -> ()  [unwired: 7 in, 3 out]
          n108 = call <vilib>:"WPI_MotorControlSetOutput.vi"("Output"=0.0, "MotorControlDevRef"=w314) -> ()  [unwired: 7 in, 3 out]
          n109 = call-poly <vilib>:"WPI_RobotDriveArcadeDrive.vi"("Y axis value"=0.0 ("X axis value"), "X axis value"=0.0, "RobotDriveDevRef"=w315) -> ()  [unwired: 1 in, 8 out]
          n110 = call <vilib>:"WPI_MotorControlSetOutput.vi"("Output"=0.0, "MotorControlDevRef"=w313) -> ()  [unwired: 7 in, 3 out]
        }
      }
    }
  }
